vi "Load Transitions.vi"(6 "Constants":refnum<class "Sequence Constants.lvclass">, 8 "error in":refnum<class "MultiErrors.lvclass">, 10 "Config Element":refnum<class "Config Element.lvclass">) -> (0 "error out":refnum<class "MultiErrors.lvclass">, 2 "Transitions":refnum<class "Transition Config.lvclass">[](array[class]))   [LabVIEW 2020, in "VolatusSeqConfig.lvlib" / "Sequence Config.lvclass"]
uses:
  Sequence Config.lvclass
  lv-cdm/CDM-Config/Config Element/Config Element.lvclass
  Transition Config/Transition Config.lvclass
  VolatusErrorUtilities/MultiErrors/MultiErrors.lvclass
  VolatusErrorUtilities/MultiErrors/MultiErrors.lvclass/MultiErrors.ctl
  Sequence Config.lvclass/Sequence Config.ctl
  VolatusSeqConfig.lvlib
  Sequence Constants/Sequence Constants.lvclass
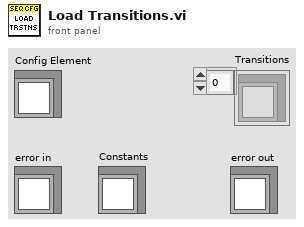
[diagram p1: front panel]
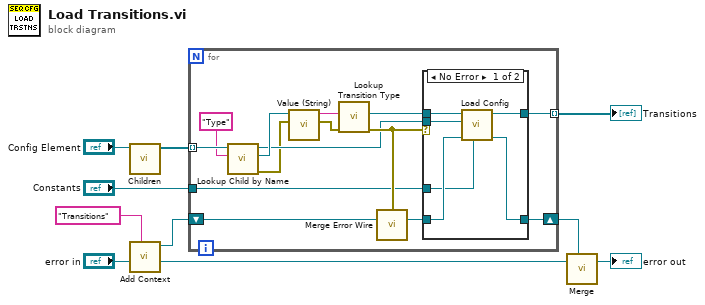
[diagram p0: block diagram]
diagram:
  n1 = call "Children.vi"("Config Element in"="Config Element") -> ("Elements"=w9:refnum<class "Config Element.lvclass">[])  [unwired: 9 in, 1 out]
  n2 = call "Add Context.vi"("Context"="Transitions", "MultiErrors in"="error in") -> ("Original Context"=w5:refnum<class "MultiErrors.lvclass">, "Added Context"=w3:refnum<class "MultiErrors.lvclass">)  [unwired: 8 in]
  n3 = for {
    tunnel: w9 -> [w23] mode=indexing
    tunnel: [w16] -> w8 mode=indexing
    shift-right: [w12] -> w2
    shift-left: w3 -> [w14]
    tunnel: "Constants" -> [w11]
    n4 = call "Lookup Child by Name.vi"("Name"="Type", "Config Element in"=w23) -> ("error out"=w15:errorcluster, "Child"=w21:refnum<class "Config Element.lvclass">, "Config Element out"=w17:refnum<class "Config Element.lvclass">)  [unwired: 6 in, 1 out]
    n5 = call "Value (String).vi"("error in (no error)"=w15, "Config Element in"=w21) -> ("error out"=w19:errorcluster, "String Value"=w20:string)  [unwired: 8 in]
    n6 = call "Lookup Transition Type.vi"("error in (no error)"=w19, "Transition Type"=w20) -> ("error out"=w24:errorcluster, "Transition"=w18:refnum<class "Transition Config.lvclass">)  [unwired: 8 in]
    n7 = call "Merge Error Wire.vi"("error in (no error)"=w24, "MultiErrors in"=w14) -> ("MultiErrors out"=w13:refnum<class "MultiErrors.lvclass">)  [unwired: 13 in]
    n8 = case shown="No Error" w24 {
      tunnel: w18 -> [w30 _]
      tunnel: w17 -> [w29 _]
      tunnel: [w28 _] -> w16
      tunnel: w13 -> [w27 w31]
      tunnel: [w26 w31] -> w12
      tunnel: w11 -> [w25 _]
      frame No Error {
        n9 = call "Load Config.vi"("Constants"=w25, "error in (no error)"=w27, "Config Element"=w29, "Transition Config in"=w30) -> ("error out"=w26:refnum<class "MultiErrors.lvclass">, "Transition Config out"=w28:refnum<class "Transition Config.lvclass">)  [unwired: 6 in]
      }
      frame Error {
      }
    }
  }
  "Transitions" <- w8
  n10 = call "Merge.vi"("First Error In"=w5, "Second Error In"=w2) -> ("MultiErrors out"=→"error out":refnum<class "MultiErrors.lvclass">)  [unwired: 5 in]
